vi "Stop Helper Loop.vi"(8 "error in (no error)":errorcluster, 9 "timeout in ms (-1)":i32=-1, 11 "Helper Loop In":refnum<class "Helper Loop.lvclass">) -> (0 "error out":errorcluster, 1 "timed out?":bool, 3 "Helper Loop Out":refnum<class "Helper Loop.lvclass">)   [LabVIEW 2020, in "Helper Loop.lvclass"]
doc: "This method stops the helper loop.The Helper Action may stop the helper loop by throwing an error. If this has happened prior to calling this method, a time out will occur."
uses:
  Helper Loop.lvclass
  Process/Process.lvclass
  <vilib>/Utility/error.llb/Error Cluster From Error Code.vi
  <vilib>/ErrorRing/Error Ring.xnode
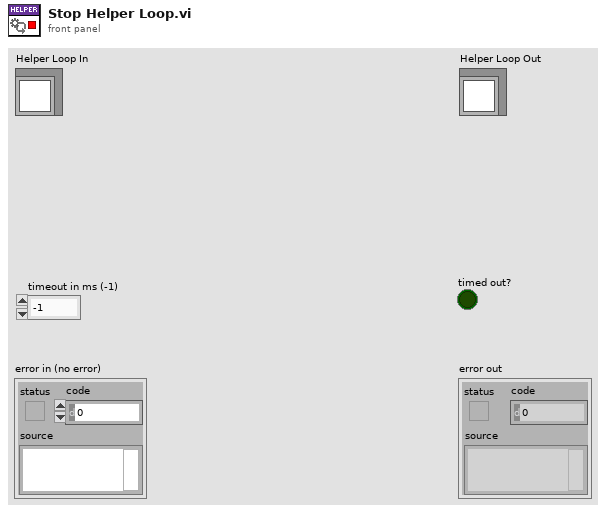
[diagram p1: front panel]
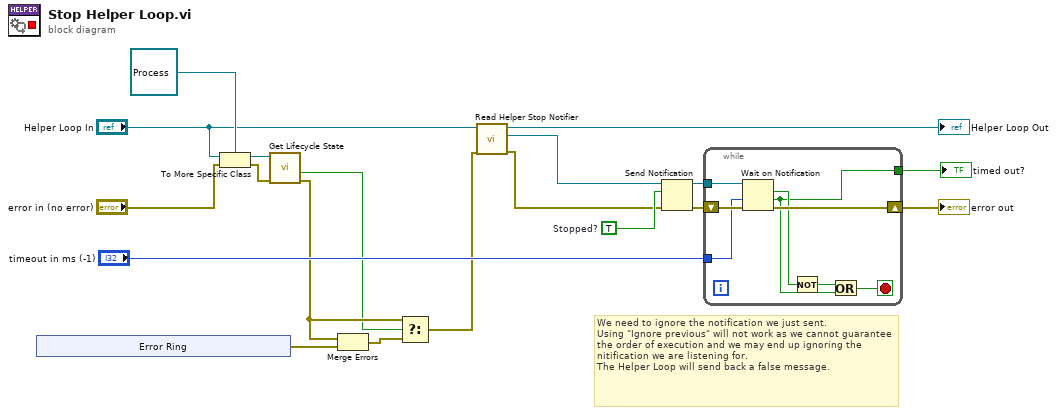
[diagram p0: block diagram]
diagram:
  w17 = TRUE  # Stopped?
  # "We need to ignore the notification we just sent. \nUsing \"Ignore previous\" will not work as we cannot guarantee the order of execution and we may end up ignoring the nitification we are listening for.\nThe Helper Loop will send back a false message."
  n1 = xnode "Error Ring"() -> ("error out"=w4:errorcluster)
  n2 = To More Specific Class(target class=refnum<class "Process.lvclass"> refnum ("Process Out"), reference="Helper Loop In", error in="error in (no error)") -> (specific class reference=w10:refnum<class "Process.lvclass">, error out=w8:errorcluster)
  n3 = call "Get Lifecycle State.vi"("error in (no error)"=w8, "Process In"=w10) -> ("error out"=w7:errorcluster, "In Process Loop?"=w6:bool)  [unwired: 6 in, 2 out]
  n4 = Merge Errors(w7, w4) -> (w5:errorcluster)
  n5 = Select(t=w7, s=w6, f=w5) -> (s? t:f=w1:errorcluster)
  n6 = call-dynamic "Read Helper Stop Notifier.vi"("error in (no error)"=w1, "Helper Loop In"="Helper Loop In") -> ("error out"=w12:errorcluster, "Helper Stopped Notifier"=w16:refnum<notifier>, "Helper Loop Out"=→"Helper Loop Out":refnum<class "Helper Loop.lvclass">)  [unwired: 7 in]
  n7 = Send Notification(notification=w17, notifier=w16, error in (no error)=w12) -> (notifier out=w11:refnum<notifier>, error out=w18:errorcluster)
  n8 = while {
    tunnel: [w20] -> w14
    tunnel: "timeout in ms (-1)" -> [w25]
    shift-right: [w26] -> w15
    shift-left: w18 -> [w27]
    tunnel: w11 -> [w21]
    stop <- w22 stop-if-true
    n9 = Wait on Notification(notifier=w21, timeout in ms (-1)=w25, error in (no error)=w27) -> (notification=w24:bool, timed out?=w20:bool, error out=w26:errorcluster)  [unwired: 1 in, 1 out]
    n10 = Not(x=w24) -> (.not. x?=w23:bool)
    n11 = Or(x=w23, y=w20) -> (x .or. y?=w22:bool)
  }
  "error out" <- w15
  "timed out?" <- w14
